vi "DelayGenerator-FringeScannerOffset.vi"(8 "error in (no error)":errorcluster, 11 "Time Stamp":timestamp) -> (0 "error out":errorcluster, 3 "DelayTarget":T1)   [LabVIEW 2009]
uses:
  Controls/DelayTarget.ctl
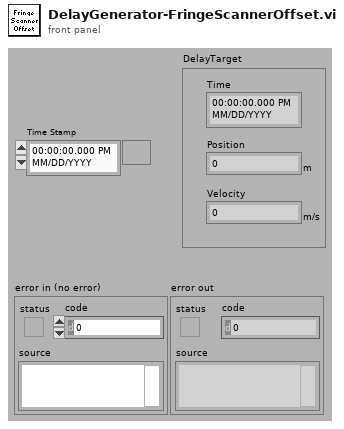
[diagram p1: front panel]
types:
  T1 = typedef "DelayTarget.ctl" = cluster{"Time":timestamp, "Position":dbl[unit], "Velocity":dbl[unit]}
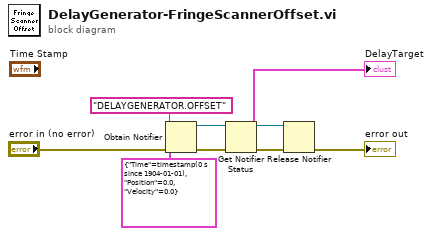
[diagram p0: block diagram]
diagram:
  n1 = Obtain Notifier(name (unnamed)="DELAYGENERATOR.OFFSET", notification data type=T1 {"Time"=timestamp(0 s since 1904-01-01), "Position"=0.0, "Velocity"=0.0} ("DelayTarget"), error in (no error)="error in (no error)") -> (notifier out=w8:refnum<notifier>, error out=w7:errorcluster)  [unwired: 1 in, 1 out]
  n2 = Get Notifier Status(notifier=w8, error in (no error)=w7) -> (notifier out=w6:refnum<notifier>, current notification=→"DelayTarget":T1, error out=w5:errorcluster)  [unwired: 2 out]
  n3 = Release Notifier(notifier=w6, error in (no error)=w5) -> (error out=→"error out":errorcluster)  [unwired: 1 in, 2 out]
